vi "SetDigitalPosition.vi"(8 "Position":i32, 10 "Controller Channel":i32, 11 "Handle":u32) -> (3 "FT_Status":u32(ring) items=["FT_OK", "FT_INVALID_HANDLE", "FT_DEVICE_NOT_FOUND", "FT_DEVICE_NOT_OPENED", "FT_IO_ERROR", "FT_INSUFFICIENT_RESOURCES", "FT_INVALID_PARAMETER", "FT_INVALID_BAUD_RATE", "FT_DEVICE_NOT_OPENED_FOR_ERASE", "FT_DEVICE_NOT_OPENED_FOR_WRITE", "FT_FAILED_TO_WRITE_DEVICE", "FT_EEPROM_READ_FAILED", "FT_EEPROM_WRITE_FAILED", "FT_EEPROM_ERASE_FAILED", "FT_EEPROM_NOT_PRESENT", "FT_EEPROM_NOT_PROGRAMMED", "FT_INVALID_ARGS", "FT_NOT_SUPPORTED", "FT_OTHER_ERROR"])   [LabVIEW 2013]
panel:
  out "Bytes Written":u32
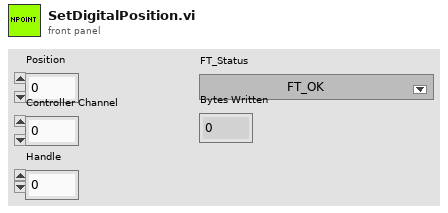
[diagram p1: front panel]
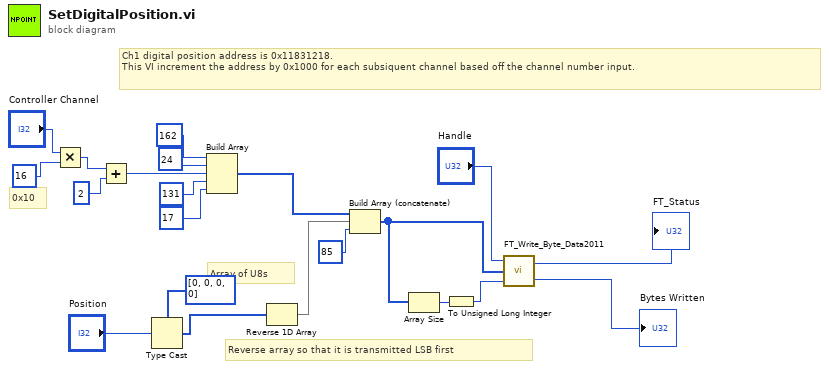
[diagram p0: block diagram]
diagram:
  # "Ch1 digital position address is 0x11831218.\nThis VI increment the address by 0x1000 for each subsiquent channel based off the channel number input."
  # "Reverse array so that it is transmitted LSB first"
  # "0x10"
  # "Array of U8s"
  n1 = Multiply(x="Controller Channel", y=u8 16) -> (x*y=w3:i32)
  n2 = Add(x=w3, y=u8 2 ("element")) -> (x+y=w2:i32)
  n3 = Type Cast(type=u8[] [0, 0, 0, 0], x="Position") -> (*(type *) &x=w11:u8[])
  n4 = Build Array(u8 162 ("element"), u8 24 ("element"), w2, u8 131 ("element"), u8 17 ("element")) -> (w14:i32[])
  n5 = Reverse 1D Array(array=w11) -> (reversed array=w10:u8[])
  n6 = Build Array (concatenate)(w14, w10, u8 85 ("element")) -> (w12:i32[])
  n7 = Array Size(array=w12) -> (size(s)=w21:i32)
  n8 = To Unsigned Long Integer(number=w21) -> (unsigned 32bit integer=w20:u32)
  n9 = call "FT_Write_Byte_Data2011.vi"("Bytes To Write"=w20, "Buffer"=w12, "Handle"="Handle") -> ("Bytes Written"=→"Bytes Written":u32, "FT_Status"=→"FT_Status":u32)
